vi "Convert Error Response to Error Cluster.vi"(10 "Error response":T1) -> (2 "error out":errorcluster)   [LabVIEW 2021]
uses:
  dcvmDPI_AD7606B_client/RPC Messages/dcvmDPI_ErrorResponse.ctl
  dcvmDPI_AD7606B_client/dcvmDPI_AD7606B_client.lvlib
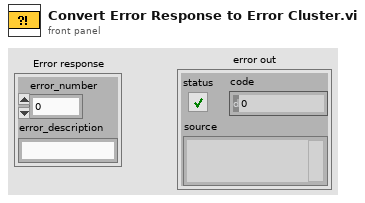
[diagram p1: front panel]
types:
  T1 = typedef "dcvmDPI_AD7606B_client.lvlib/dcvmDPI_ErrorResponse.ctl" = cluster{"error_number":i32, "error_description":string}
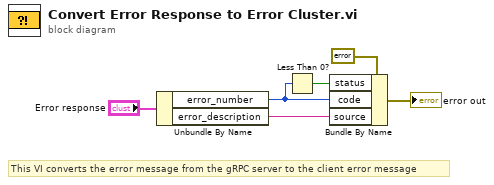
[diagram p0: block diagram]
diagram:
  # "This VI converts the error message from the gRPC server to the client error message"
  n1 = Unbundle By Name("Error response") -> ("error_number"=w2:i32, "error_description"=w4:string)
  n2 = Less Than 0?(x=w2) -> (x < 0?=w3:bool)
  n3 = Bundle By Name(cluster=errorcluster {"status"=FALSE, "code"=0, "source"=""} ("error out"), "status"=w3, "code"=w2, "source"=w4) -> (→"error out":errorcluster)
